vi "Center2.vi"(6 "Pretrigger Samples?":i32, 7 "Not enough Data?":bool=TRUE, 8 "error in (no error)":errorcluster, 9 "Num Samples":dbl, 10 "Data In":dbl[][](array[numeric]), 11 "DAQmx Task In":refnum<k21>) -> (0 "error out":errorcluster, 2 "Data Out":dbl[][](array[numeric]), 3 "DAQmx Task Out":refnum<k21>)   [LabVIEW 2013]
uses:
  <vilib>/_DAQmxBase/Internals/DAQmxBase Read (Analog 2D DBL NChan NSamp).vi
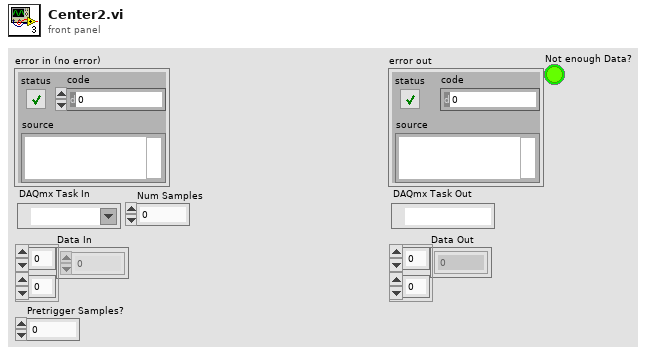
[diagram p1: front panel]
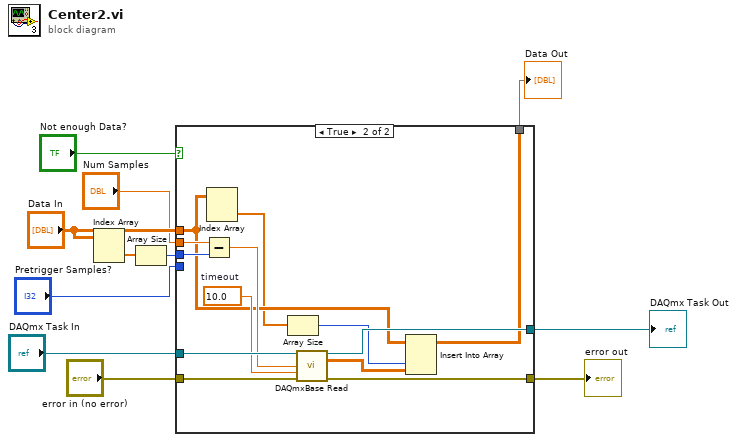
[diagram p0: block diagram]
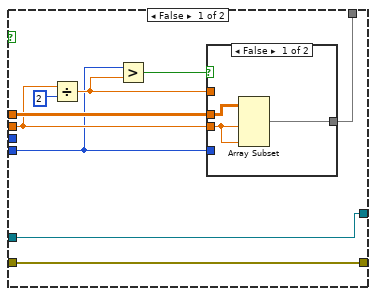
[diagram p2: hidden frame]
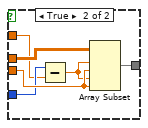
[diagram p3: hidden frame]
diagram:
  n1 = Index Array(array="Data In") -> (element=w4:dbl[])  [unwired: 2 in]
  n2 = Array Size(array=w4) -> (size(s)=w3:i32)
  n3 = case shown="True" "Not enough Data?" {
    tunnel: "error in (no error)" -> [w19 w42]
    tunnel: [w19 w41] -> w10
    tunnel: "DAQmx Task In" -> [w20 w40]
    tunnel: [w20 w39] -> w8
    tunnel: "Num Samples" -> [w14 w35]
    tunnel: "Data In" -> [w18 w31]
    tunnel: [w17 w34] -> w7
    tunnel: w3 -> [_ w36]
    tunnel: "Pretrigger Samples?" -> [w12 _]
    frame False {
      n4 = Divide(x=w14, y=2) -> (x/y=w13:dbl)
      n5 = Greater?(x=w12, y=w13) -> (0:w16:bool)
      n6 = case shown="False" w16 {
        tunnel: w18 -> [w23 w29]
        tunnel: [w22 w28] -> w17
        tunnel: w14 -> [w21 w27]
        tunnel: w13 -> [_ w25]
        tunnel: w12 -> [_ w26]
        frame False {
          n7 = Array Subset(array=w23, length (row)=w21, length (col)=w21) -> (w22:dbl[][])  [unwired: 2 in]
        }
        frame True {
          n8 = Subtract(x=w26, y=w25) -> (x-y=w24:dbl)
          n9 = Array Subset(array=w29, index (row)=w24, length (row)=w27, index (col)=w24, length (col)=w27) -> (w28:dbl[][])
        }
      }
    }
    frame True {
      w38 = 10.0  # timeout
      n10 = Subtract(x=w35, y=w36) -> (x-y=w37:dbl)
      n11 = Index Array(array=w31) -> (element=w30:dbl[])  [unwired: 2 in]
      n12 = Array Size(array=w30) -> (size(s)=w32:i32)
      n13 = call-poly <vilib>:"DAQmxBase Read.vi"("task/channels in"=w40, "number of samples per channel"=w37, "timeout"=w38, "error in"=w42) -> ("task out"=w39:refnum<k21>, "data"=w33:dbl[][], "error out"=w41:errorcluster)  [unwired: 9 in]
      n14 = Insert Into Array(array=w31, index (col)=w32, new element=w33) -> (w34:dbl[][])  [unwired: 1 in]
    }
  }
  "error out" <- w10
  "DAQmx Task Out" <- w8
  "Data Out" <- w7
